vi "Introspection Core.vi"(8 "error in (no error)":errorcluster, 11 "CS++FgenGui in":refnum<class "CS++FgenGui.lvclass">) -> (0 "error out":errorcluster, 2 "CS++Messages":refnum<class "Message.lvclass">[](array[class]), 3 "CS++FgenGui out":refnum<class "CS++FgenGui.lvclass">)   [LabVIEW 2014, in "CS++FgenGui.lvlib" / "CS++FgenGui.lvclass"]
doc: "This vi delivers a list with all messages this actor reacts to. \n\nNote that all inherited classes have to overwrite it."
uses:
  CS++FgenGui.lvclass
  <vilib>/ActorFramework/Message/Message.lvclass
  CS++DCPwrGui Messages/Update PV Msg/Update PV Msg.lvclass
  CSPP_Core/Actors/CS++DeviceGUIActor/CS++DeviceGUIActor.lvclass
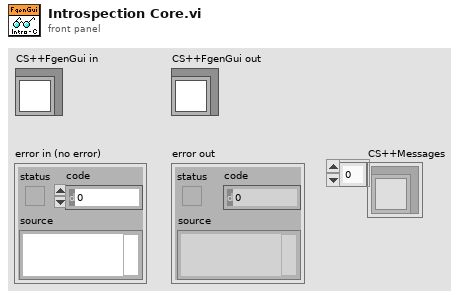
[diagram p1: front panel]
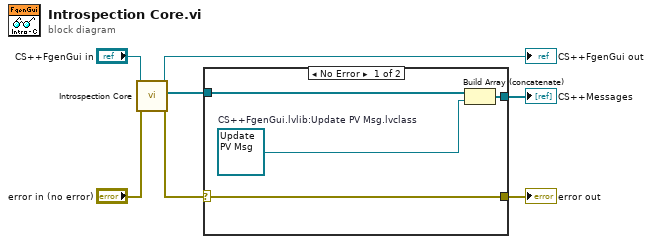
[diagram p0: block diagram]
diagram:
  n1 = call-parent "Introspection Core.vi"("error in (no error)"="error in (no error)", "CS++DeviceGUIActor in"="CS++FgenGui in") -> ("error out"=w4:errorcluster, "CS++Messages"=w2:refnum<class "Message.lvclass">[], "CS++DeviceGUIActor out"=→"CS++FgenGui out":refnum<class "CS++FgenGui.lvclass">)  [unwired: 7 in]
  n2 = case shown="No Error" w4 {
    selector: w4 -> [w11 w12]
    tunnel: [w11 w12] -> w3
    tunnel: w2 -> [w10 _]
    tunnel: [w8 _] -> w1
    frame No Error {
      w9 = refnum<class "Update PV Msg.lvclass"> refnum  # CS++FgenGui.lvlib:Update PV Msg.lvclass
      n3 = Build Array (concatenate)(w10, w9) -> (w8:refnum<class "Message.lvclass">[])
    }
    frame Error {
    }
  }
  "error out" <- w3
  "CS++Messages" <- w1
